vi "SMU Reset.vi"(8 "error in (no error)":errorcluster, 9 "Remote Node (1)":i32=1, 10 "Reset Module (0: Entire System)":i32(ring) items=["Entire System", "Local Group", "Local Node", "Remote Node", "Source Measure Unit Channel A", "Source Measure Unit Channel B", "LAN", "TSP Net", "TSP Link", "Timer"], 11 "VISA resource name":refnum<visa-resource-name>) -> (0 "error out":errorcluster, 3 "VISA resource name out":refnum<visa-resource-name>)   [LabVIEW 2019, in "Keithley 2600 Series.lvlib"]
doc: "Recalls factory default setting."
uses:
  <instrlib>/Keithley 2600 Series/Keithley 2600 Series.lvlib
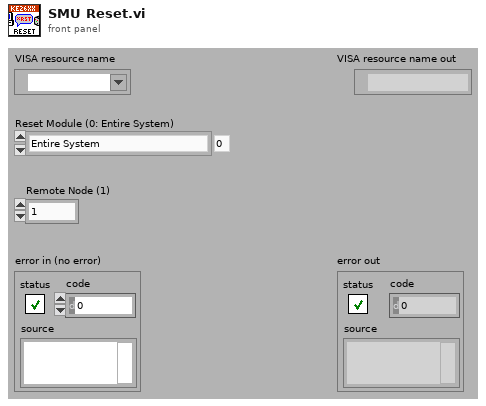
[diagram p1: front panel]
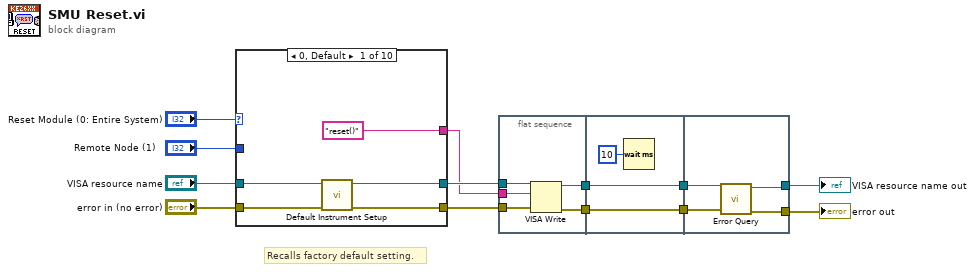
[diagram p0: block diagram]
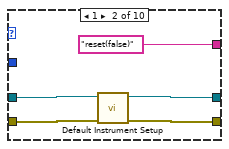
[diagram p2: hidden frame]
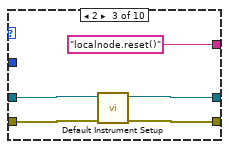
[diagram p3: hidden frame]
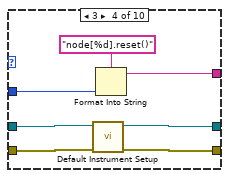
[diagram p4: hidden frame]
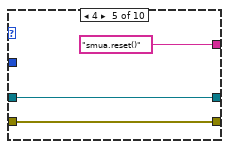
[diagram p5: hidden frame]
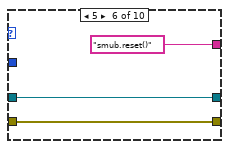
[diagram p6: hidden frame]
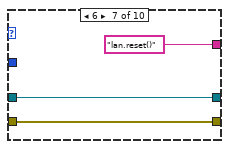
[diagram p7: hidden frame]
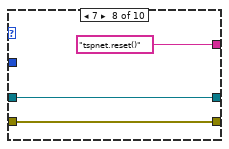
[diagram p8: hidden frame]
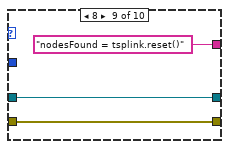
[diagram p9: hidden frame]
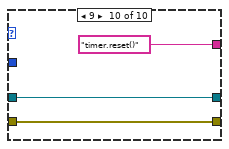
[diagram p10: hidden frame]
diagram:
  # "Recalls factory default setting."
  n1 = case shown="0, Default" "Reset Module (0: Entire System)" {
    tunnel: ["reset()" "reset(false)" "localnode.reset()" w35 "smua.reset()" "smub.reset()" "lan.reset()" "tspnet.reset()" "nodesFound = tsplink.reset()" "timer.reset()"] -> w8
    tunnel: "Remote Node (1)" -> [_ _ _ w33 _ _ _ _ _ _]
    tunnel: "VISA resource name" -> [w14 w22 w27 w32 w37 w40 w43 w46 w49 w52]
    tunnel: "error in (no error)" -> [w17 w21 w26 w31 w36 w39 w42 w45 w48 w51]
    tunnel: [w16 w20 w25 w30 w37 w40 w43 w46 w49 w52] -> w9
    tunnel: [w15 w19 w24 w29 w36 w39 w42 w45 w48 w51] -> w7
    frame 0, Default {
      n2 = call <instrlib>:"Default Instrument Setup.vi"("error in (no error)"=w17, "VISA resource name"=w14) -> ("error out"=w15:errorcluster, "VISA resource name out"=w16:refnum<visa-resource-name>)  [unwired: 8 in]
    }
    frame 1 {
      n3 = call <instrlib>:"Default Instrument Setup.vi"("error in (no error)"=w21, "VISA resource name"=w22) -> ("error out"=w19:errorcluster, "VISA resource name out"=w20:refnum<visa-resource-name>)  [unwired: 8 in]
    }
    frame 2 {
      n4 = call <instrlib>:"Default Instrument Setup.vi"("error in (no error)"=w26, "VISA resource name"=w27) -> ("error out"=w24:errorcluster, "VISA resource name out"=w25:refnum<visa-resource-name>)  [unwired: 8 in]
    }
    frame 3 {
      n5 = call <instrlib>:"Default Instrument Setup.vi"("error in (no error)"=w31, "VISA resource name"=w32) -> ("error out"=w29:errorcluster, "VISA resource name out"=w30:refnum<visa-resource-name>)  [unwired: 8 in]
      n6 = Format Into String(format string="node[%d].reset()", w33) -> (resulting string=w35:string)  [unwired: 2 in, 1 out]
    }
    frame 4 {
    }
    frame 5 {
    }
    frame 6 {
    }
    frame 7 {
    }
    frame 8 {
    }
    frame 9 {
    }
  }
  n7 = flat-sequence {
    tunnel: w9 -> [w58]
    tunnel: w8 -> [w57]
    tunnel: w7 -> [w56]
    tunnel: [w55] -> w6
    tunnel: [w54] -> w4
    tunnel: w6 -> [w61]
    tunnel: [w61] -> w5
    tunnel: w4 -> [w60]
    tunnel: [w60] -> w3
    tunnel: w5 -> [w63]
    tunnel: [w62] -> w1
    tunnel: w3 -> [w65]
    tunnel: [w64] -> w2
    frame #0 {
      n8 = VISA Write(VISA resource name=w58, write buffer=w57, error in (no error)=w56) -> (VISA resource name out=w55:refnum<visa-resource-name>, error out=w54:errorcluster)  [unwired: 1 out]
    }
    frame #1 {
      n9 = Wait (ms)(milliseconds to wait=u32 10) -> ()  [unwired: 1 out]
    }
    frame #2 {
      n10 = call <instrlib>:"Error Query.vi"("error in (no error)"=w65, "VISA resource name"=w63) -> ("error out"=w64:errorcluster, "VISA resource name out"=w62:refnum<visa-resource-name>)  [unwired: 6 in, 2 out]
    }
  }
  "VISA resource name out" <- w1
  "error out" <- w2
